vi "set_params.vi"(8 "error in (no error)":errorcluster caption="entrée d'erreur (pas d'erreur)", 11 "MLPClassifier.lvclass 2":refnum<class "MLPClassifier.lvclass">) -> (0 "error out":errorcluster caption="sortie d'erreur", 3 "MLPClassifier.lvclass":refnum<class "MLPClassifier.lvclass">)   [LabVIEW 2020, in "MLPClassifier.lvclass"]
uses:
  MLPClassifier.lvclass
  MLPClassifier.lvclass/MLPClassifier.ctl
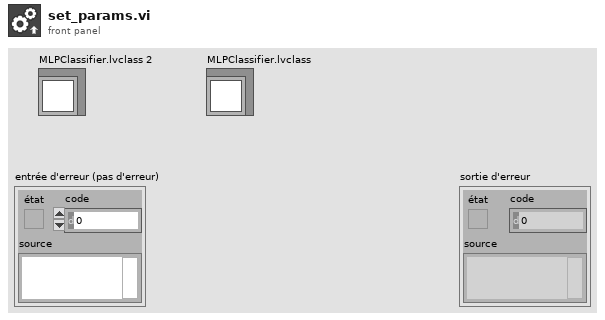
[diagram p1: front panel]
types:
  T1 = typedef "mlp_classifier_params.ctl" = cluster{"hidden_layer_sizes":dbl[], "activation":string, "solver":string, "alpha":dbl, "batch_size":cluster{"batch_size_type":string, "batch_size_int":dbl}, "learning_rate":string, "learning_rate_init":dbl, "power_t":dbl, "max_iter":dbl, "shuffle":bool, "random_state":dbl, "tol":dbl, "verbose":bool, "warm_start":bool, "momentum":dbl, "nesterovs_momentum":bool, "early_stopping":bool, "validation_fraction":dbl, "beta_1":dbl, "beta_2":dbl, "epsilon":dbl, "n_iter_no_change":dbl, "max_fun":dbl}
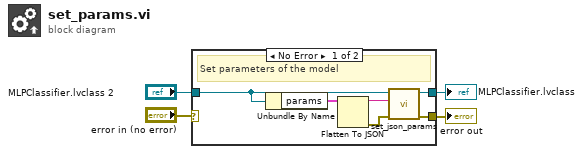
[diagram p0: block diagram]
diagram:
  n1 = case shown="No Error" "error in (no error)" {
    selector: "error in (no error)" -> [_ w12]
    tunnel: [w7 w12] -> w3
    tunnel: [w8 w11] -> w1
    tunnel: "MLPClassifier.lvclass 2" -> [w5 w11]
    frame No Error {
      # "Set parameters of the model"
      n2 = Unbundle By Name(w5) -> ("params"=w10:T1)
      n3 = Flatten To JSON(anything=w10) -> (JSON string=w9:string, 11:w6:errorcluster)  [unwired: 2 in]
      n4 = call-dynamic "set_json_params.vi"("error in (no error)"=w6, "params"=w9, "Model en entrée"=w5) -> ("error out"=w7:errorcluster, "Model en sortie"=w8:refnum<class "MLPClassifier.lvclass">)  [unwired: 7 in]
    }
    frame Error {
    }
  }
  "error out" <- w3
  "MLPClassifier.lvclass" <- w1
